vi "loadLut.vi"(8 "error in (no error)":errorcluster, 9 "lut_file":path, 10 "data_format":T1(ring)=enum."Mono16", 11 "Camera in":refnum<class "Camera.lvclass">) -> (0 "error out":errorcluster, 3 "Camera out":refnum<class "Camera.lvclass">)   [LabVIEW 2019, in "Camera.lvclass"]
doc: "Loads a Lookup Table (LUT) from a flie. LUT's are used to apply pseudocolor to monochrome images."
uses:
  Camera.lvclass
  Camera.lvclass/Camera.ctl
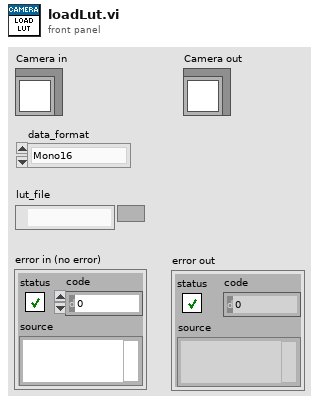
[diagram p1: front panel]
types:
  T1 = enum16{"Undefined", "Mono8", "Mono16", "BGRA8", "RGBA8", "BGRA16", "RGBA16", "CompressedMono8"}
  T2 = map{enum16{"Undefined", "Mono8", "Mono16", "RGB8", "RGBA8", "RGB16", "CompressedMono8"}, u64}
  T3 = map{enum16{"Undefined", "Mono8", "Mono16", "BGRA8", "RGBA8", "BGRA16", "RGBA16", "CompressedMono8"}, cluster{"sharpen":bool, "adaptive_sharpen":bool, "flip_vertical":bool, "auto_minmax":bool, "add_conv_flags":u32, "min_limit":u16, "max_limit":u16, "gamma":dbl, "contrast":i32, "pco_debayer_algorithm":bool, "color_temperature":i32, "color_saturation":i32, "color_vibrance":i32, "color_tint":i32, "lut_file":path}}
  T4 = cluster{"sharpen":bool, "adaptive_sharpen":bool, "flip_vertical":bool, "auto_minmax":bool, "add_conv_flags":u32, "min_limit":u16, "max_limit":u16, "gamma":dbl, "contrast":i32, "pco_debayer_algorithm":bool, "color_temperature":i32, "color_saturation":i32, "color_vibrance":i32, "color_tint":i32, "lut_file":path}
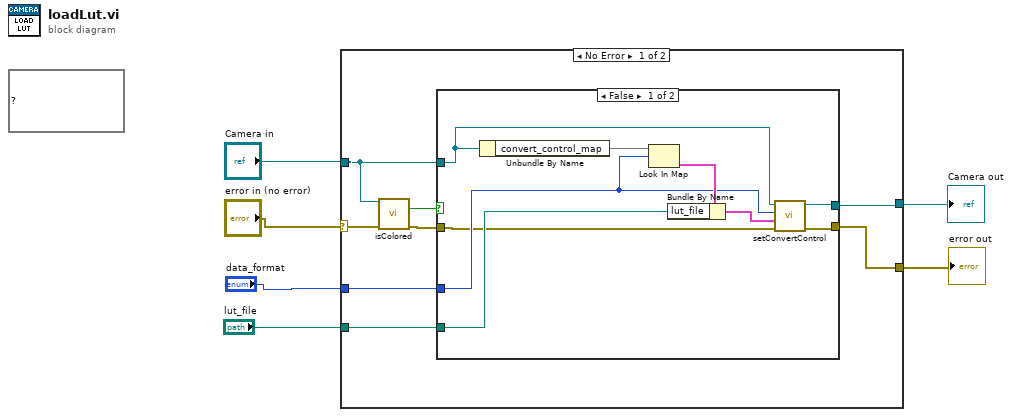
[diagram p0: block diagram]
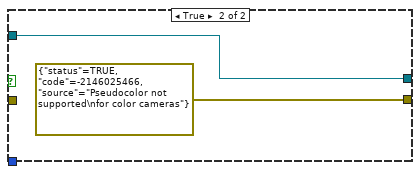
[diagram p2: hidden frame]
diagram:
  (unwired) T2 {} ("convert_handles")
  n1 = case shown="No Error" "error in (no error)" {
    selector: "error in (no error)" -> [w12 w27]
    tunnel: [w8 w27] -> w4
    tunnel: [w7 w26] -> w5
    tunnel: "Camera in" -> [w11 w26]
    tunnel: "lut_file" -> [w9 _]
    tunnel: "data_format" -> [w10 _]
    frame No Error {
      n2 = call-dynamic "isColored.vi"("Camera in"=w11, "error in (no error)"=w12) -> ("colored"=w13:bool, "error out"=w14:errorcluster)  [unwired: 11 in, 1 out]
      n3 = case shown="False" w13 {
        tunnel: w14 -> [w17 _]
        tunnel: [w16 errorcluster {"status"=TRUE, "code"=-2146025466, "source"="Pseudocolor not supported\nfor color cameras"} ("error IO")] -> w8
        tunnel: w11 -> [w18 w24]
        tunnel: w10 -> [w19 _]
        tunnel: w9 -> [w22 _]
        tunnel: [w15 w24] -> w7
        frame False {
          n4 = Unbundle By Name(w18) -> ("convert_control_map"=w21:T3)
          n5 = Look In Map(map=w21, key=w19) -> (value=w23:T4)  [unwired: 1 in, 1 out]
          n6 = Bundle By Name(cluster=w23, "lut_file"=w22) -> (w20:T4)
          n7 = call-dynamic "setConvertControl.vi"("error in (no error)"=w17, "convert_control"=w20, "data_format"=w19, "Camera in"=w18) -> ("error out"=w16:errorcluster, "Camera out"=w15:refnum<class "Camera.lvclass">)  [unwired: 6 in]
        }
        frame True {
        }
      }
    }
    frame Error {
    }
  }
  "error out" <- w4
  "Camera out" <- w5
